vi "Set Speed.vi"(8 "error in (no error)":errorcluster, 10 "speed":dbl, 11 "FLOM Settings in":T1={"VISA resource name"="", "Simulated?"=FALSE, "Pump Number"=1.0} {"Pump Number" min=1.0 max=20.0 step=1.0}) -> (0 "error out":errorcluster, 1 "Connection Error":bool, 3 "FLOM Settings out":T1={"VISA resource name"="", "Simulated?"=FALSE, "Pump Number"=1.0} {"Pump Number" min=1.0 max=20.0 step=1.0})   [LabVIEW 2018, in "FLOM Pump.lvlib"]
uses:
  FLOM Pump.lvlib
  Settings Cluster.ctl
panel:
  out "read buffer":string
  out "decimal integer string":string
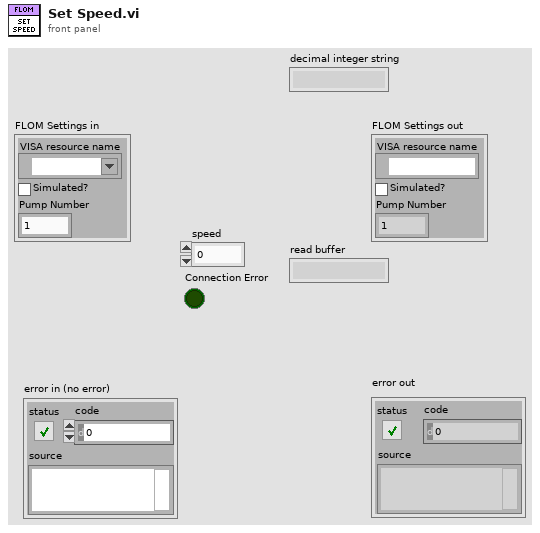
[diagram p1: front panel]
types:
  T1 = typedef "FLOM Pump.lvlib/Settings Cluster.ctl" = cluster{"VISA resource name":refnum<visa-resource-name>, "Simulated?":bool, "Pump Number":dbl}
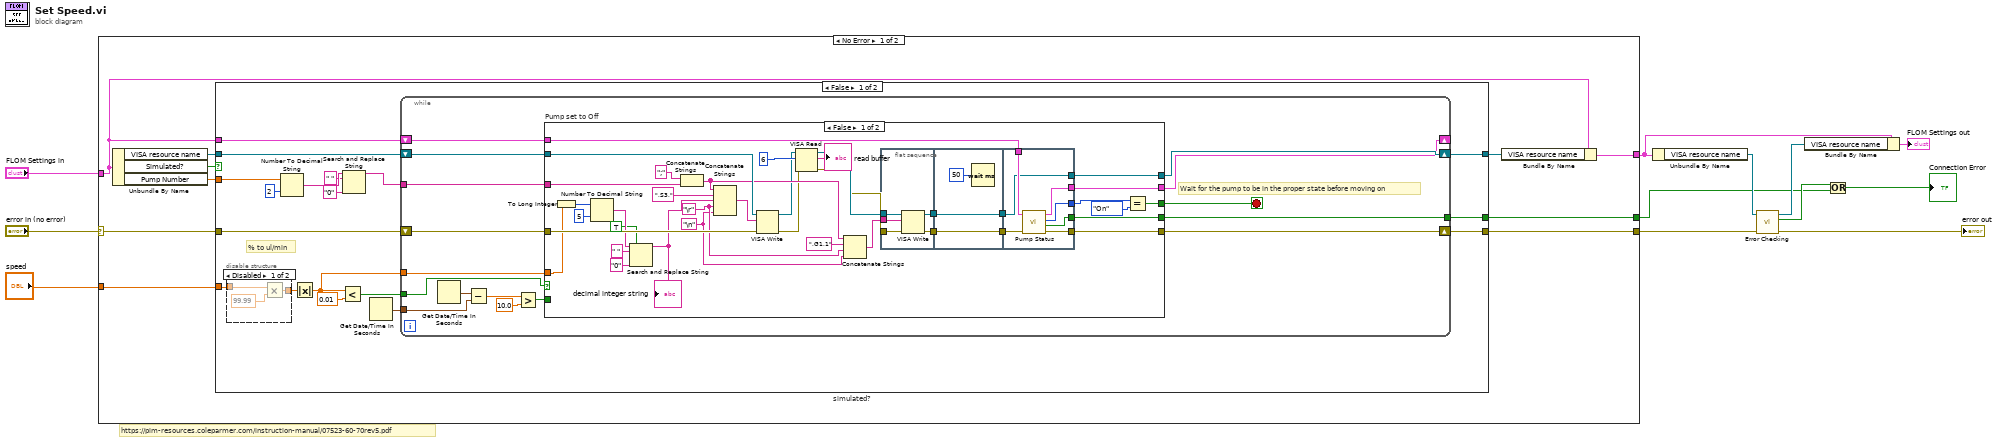
[diagram p0: block diagram]
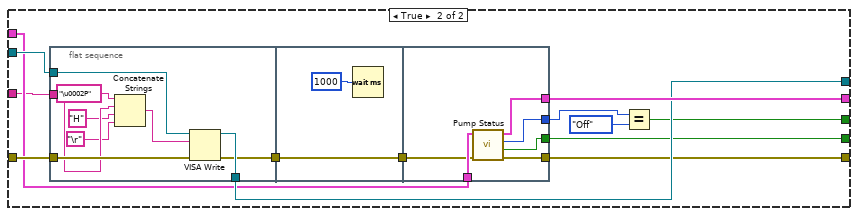
[diagram p3: hidden frame]
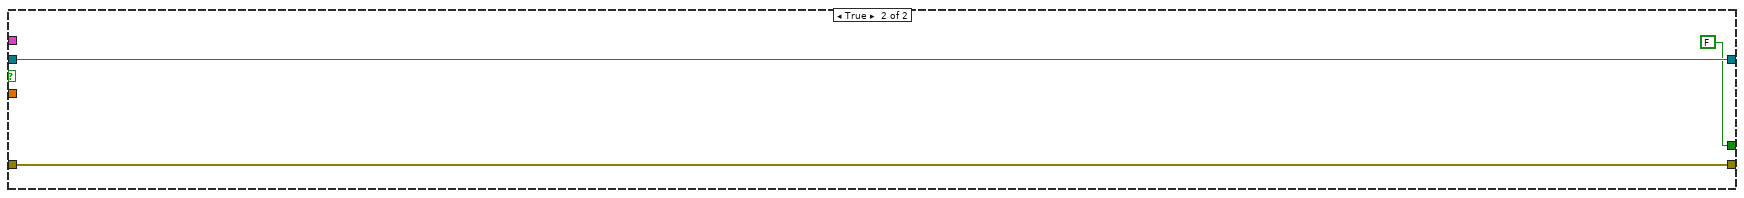
[diagram p4: hidden frame]
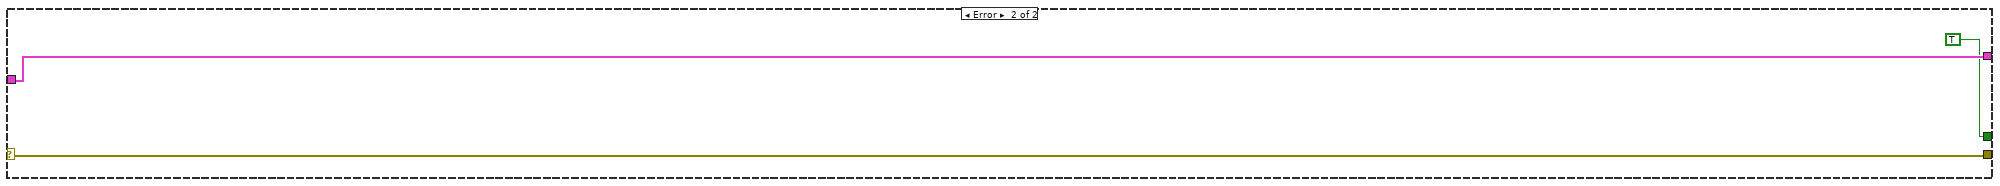
[diagram p5: hidden frame]
diagram:
  # "https://pim-resources.coleparmer.com/instruction-manual/07523-60-70rev5.pdf"
  n1 = case shown="No Error" "error in (no error)" {
    selector: "error in (no error)" -> [w20 w148]
    tunnel: [w19 w148] -> w9
    tunnel: [w17 w147] -> w7
    tunnel: "FLOM Settings in" -> [w14 w147]
    tunnel: "speed" -> [w18 _]
    tunnel: [w13 TRUE ("Connection Error")] -> w2
    frame No Error {
      n2 = Unbundle By Name(w14) -> ("VISA resource name"=w16:refnum<visa-resource-name>, "Simulated?"=w22:bool, "Pump Number"=w21:dbl)
      n3 = case "simulated?" shown="False" w22 {
        tunnel: w20 -> [w33 w145]
        tunnel: [w38 w145] -> w19
        tunnel: w21 -> [w24 _]
        tunnel: w18 -> [w35 _]
        tunnel: w16 -> [w32 w144]
        tunnel: [w34 w144] -> w15
        tunnel: w14 -> [w30 _]
        tunnel: [w29 FALSE ("Connection Error")] -> w13
        frame False {
          # "% to ul/min"
          n4 = disable-structure shown="Disabled" {
            disable-tunnel: [w42 w44] -> w37
            disable-tunnel: w35 -> [w41 w44]
            frame Disabled {
              n5 = Multiply(x=w41, y=99.99) -> (x*y=w42:dbl)
            }
            frame Enabled {
            }
          }
          n6 = Number To Decimal String(number=w24, width (-)=i16 2) -> (decimal integer string=w27:string)
          n7 = Absolute Value(x=w37) -> (abs(x)=w36:dbl)
          n8 = Less?(x=w36, y=0.01) -> (x < y?=w39:bool)
          n9 = Search and Replace String(input string=w27, search string=" ", replace string="0" ("replace string (\"\")")) -> (result string=w23:string)  [unwired: 5 in, 3 out]
          n10 = Get Date/Time In Seconds() -> (seconds since 1Jan1904=w31:timestamp)
          n11 = while {
            tunnel: w39 -> [w60]
            tunnel: w36 -> [w58]
            tunnel: w23 -> [w49]
            shift-right: [w59] -> w38
            shift-left: w33 -> [w51]
            shift-right: [w57] -> w34
            shift-left: w32 -> [w50]
            tunnel: w31 -> [w53]
            shift-right: [w52] -> _
            shift-left: w30 -> [w48]
            tunnel: [w47] -> w29
            stop <- w45 stop-if-true
            # "Wait for the pump to be in the proper state before moving on"
            n12 = Get Date/Time In Seconds() -> (seconds since 1Jan1904=w56:timestamp)
            n13 = Subtract(x=w56, y=w53) -> (x-y=w54:dbl)
            n14 = Greater?(x=w54, y=10.0) -> (0:w46:bool)
            n15 = case "Pump set to Off" shown="False" w60 {
              tunnel: [w91 w119] -> w59
              tunnel: w58 -> [w63 _]
              tunnel: [w92 w121] -> w57
              tunnel: w49 -> [w79 w117]
              tunnel: w46 -> [_ _]
              tunnel: w48 -> [w90 w118]
              tunnel: [w89 w124] -> w52
              tunnel: w51 -> [w87 w125]
              tunnel: w50 -> [w88 w120]
              tunnel: [w86 w116] -> w47
              tunnel: [w83 w113] -> w45
              frame False {
                w75 = "\n"
                w76 = "\r"
                n16 = To Long Integer(number=w63) -> (32bit integer=w62:i32)
                n17 = Number To Decimal String(number=w62, width (-)=i16 5) -> (decimal integer string=w65:string)
                n18 = Search and Replace String(replace all?=TRUE ("replace all? (F)"), input string=w65, search string=" ", replace string="0" ("replace string (\"\")")) -> (result string=w64:string)  [unwired: 4 in, 3 out]
                "decimal integer string" <- w64
                n19 = Concatenate Strings(";" ("string"), w79) -> (w78:string)
                n20 = Concatenate Strings(w78, ",S3," ("string"), w64, w76, w75) -> (w97:string)
                n21 = VISA Write(VISA resource name=w88, write buffer=w97, error in (no error)=w87) -> (VISA resource name out=w72:refnum<visa-resource-name>, error out=w70:errorcluster)  [unwired: 1 out]
                n22 = VISA Read(VISA resource name=w72, byte count=u32 6, error in (no error)=w70) -> (VISA resource name out=w71:refnum<visa-resource-name>, read buffer=→"read buffer":string, error out=w69:errorcluster)  [unwired: 1 out]
                n23 = Concatenate Strings(w78, ",G1,1" ("string"), w76, w75) -> (w82:string)
                n24 = flat-sequence {
                  tunnel: w69 -> [w102]
                  tunnel: w82 -> [w101]
                  tunnel: w71 -> [w100]
                  tunnel: [w99] -> w96
                  tunnel: [w98] -> w93
                  tunnel: w96 -> [w104]
                  tunnel: [w104] -> w95
                  tunnel: [w103] -> w94
                  tunnel: w93 -> [w103]
                  tunnel: w95 -> [w109]
                  tunnel: w94 -> [w111]
                  tunnel: [w109] -> w92
                  tunnel: [w110] -> w91
                  tunnel: w90 -> [w112]
                  tunnel: [w106] -> w89
                  tunnel: [w108] -> w85
                  tunnel: [w107] -> w86
                  frame #0 {
                    n25 = VISA Write(VISA resource name=w100, write buffer=w101, error in (no error)=w102) -> (VISA resource name out=w99:refnum<visa-resource-name>, error out=w98:errorcluster)  [unwired: 1 out]
                  }
                  frame #1 {
                    n26 = Wait (ms)(milliseconds to wait=u32 50) -> ()  [unwired: 1 out]
                  }
                  frame #2 {
                    n27 = call "Pump Status.vi"("error in (no error)"=w111, "FLOM Settings In"=w112) -> ("error out"=w110:errorcluster, "Connection Error"=w107:bool, "Pump On?"=w108:enum16{"Off", "On", "Not Initialized"}, "FLOM Settings Out"=w106:T1)  [unwired: 4 in, 2 out]
                  }
                }
                n28 = Equal?(x=w85, y=enum16{"Off", "On", "Not Initialized"}."On") -> (x = y?=w83:bool)
              }
              frame True {
                n29 = flat-sequence {
                  tunnel: w125 -> [w133]
                  tunnel: w120 -> [w132]
                  tunnel: w117 -> [w130]
                  tunnel: [w127] -> w121
                  tunnel: [w126] -> w122
                  tunnel: [w135] -> w123
                  tunnel: w122 -> [w135]
                  tunnel: w118 -> [w142]
                  tunnel: [w141] -> w115
                  tunnel: [w140] -> w124
                  tunnel: w123 -> [w139]
                  tunnel: [w138] -> w119
                  tunnel: [w137] -> w116
                  frame #0 {
                    n30 = Concatenate Strings("\u0002P" ("string"), w130, "H" ("string"), "\r") -> (w134:string)
                    n31 = VISA Write(VISA resource name=w132, write buffer=w134, error in (no error)=w133) -> (VISA resource name out=w127:refnum<visa-resource-name>, error out=w126:errorcluster)  [unwired: 1 out]
                  }
                  frame #1 {
                    n32 = Wait (ms)(milliseconds to wait=u32 1000) -> ()  [unwired: 1 out]
                  }
                  frame #2 {
                    n33 = call "Pump Status.vi"("error in (no error)"=w139, "FLOM Settings In"=w142) -> ("error out"=w138:errorcluster, "Connection Error"=w137:bool, "Pump On?"=w141:enum16{"Off", "On", "Not Initialized"}, "FLOM Settings Out"=w140:T1)  [unwired: 4 in, 2 out]
                  }
                }
                n34 = Equal?(x=w115, y=enum16{"Off", "On", "Not Initialized"}."Off") -> (x = y?=w113:bool)
              }
            }
          }
        }
        frame True {
        }
      }
      n35 = Bundle By Name(cluster=w14, "VISA resource name"=w15) -> (w17:T1)
    }
    frame Error {
    }
  }
  n36 = Unbundle By Name(w7) -> ("VISA resource name"=w12:refnum<visa-resource-name>)
  n37 = call "Error Checking.vi"("error in (no error)"=w9, "VISA resource name"=w12) -> ("error out"=→"error out":errorcluster, "Connection Error"=w3:bool, "VISA resource name"=w11:refnum<visa-resource-name>)  [unwired: 7 in]
  n38 = Bundle By Name(cluster=w7, "VISA resource name"=w11) -> (→"FLOM Settings out":T1)
  n39 = Or(x=w3, y=w2) -> (x .or. y?=→"Connection Error":bool)
